vi "field oriented translation.vi"(2 "x in":dbl(slide) scale=-1.0..1.0, 3 "y in":dbl(slide) scale=-1.0..1.0) -> (0 "x out":dbl(slide) scale=0.0..100.0, 1 "y out":dbl(slide) scale=0.0..100.0)   [LabVIEW 2023]
uses:
  <vilib>/Rock Robotics/WPI/ThirdParty/Phoenix-LabVIEW/Pigeon IMU/CTRE_PigeonIMU_GetYPR.vi
panel:
  out "Angle out":dbl
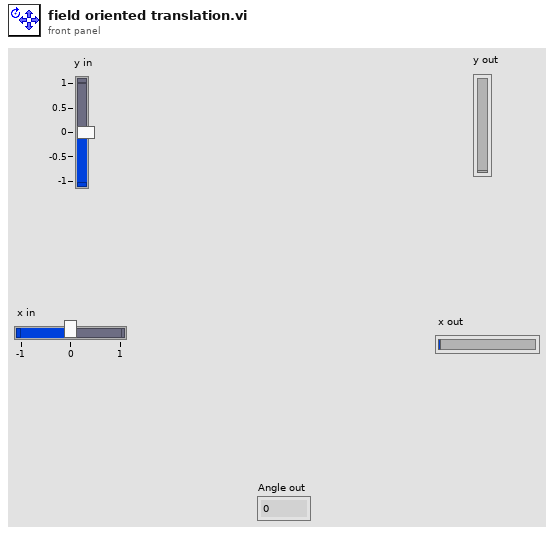
[diagram p1: front panel]
types:
  T1 = typedef "CTRE_PigeonIMU_DeviceRef.ctl" = cluster{"DeviceStatus":errorcluster, "Device Number":u8, "Type":T2, "Device ID":u32, "Handle":u64, "UsageFrame":u32, "Library Path":path}
  T2 = typedef "CTRE_PigeonIMU_ConnectionType.ctl" = u32
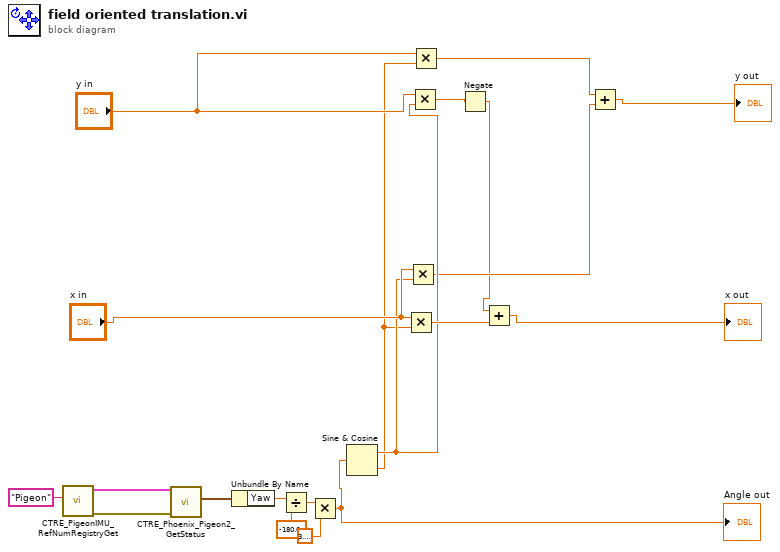
[diagram p0: block diagram]
diagram:
  n1 = call <vilib>:"CTRE_PigeonIMU_RefNumRegistryGet.vi"("refnum name"="Pigeon") -> ("error out"=w18:errorcluster, "PigeonIMUDevRef"=w19:T1)  [unwired: 9 in]
  n2 = call-poly <vilib>:"CTRE_Phoenix_Pigeon2_GetStatus.vi"("error in (no error)"=w18, "PigeonIMUDevRef"=w19) -> ("Yaw Pitch Roll"=w17:cluster{"Yaw":dbl, "Pitch":dbl, "Roll":dbl})  [unwired: 7 in, 2 out]
  n3 = Unbundle By Name(w17) -> ("Yaw"=w16:dbl)
  n4 = Divide(x=w16, y=-180.0) -> (x/y=w14:dbl)
  n5 = Multiply(x=w14, y=3.141592653589793) -> (x*y=w12:dbl)
  "Angle out" <- w12
  n6 = Sine & Cosine(0:w12) -> (1:w8:dbl, 2:w6:dbl)
  n7 = Multiply(x="x in", y=w6) -> (x*y=w11:dbl)
  n8 = Multiply(x="x in", y=w8) -> (x*y=w4:dbl)
  n9 = Multiply(x="y in", y=w8) -> (x*y=w1:dbl)
  n10 = Multiply(x="y in", y=w6) -> (x*y=w5:dbl)
  n11 = Negate(x=w1) -> (-x=w2:dbl)
  n12 = Add(x=w2, y=w11) -> (x+y=→"x out":dbl)
  n13 = Add(x=w5, y=w4) -> (x+y=→"y out":dbl)
